vi "Set Instrument Addon Name.vi"(8 "Error In":errorcluster, 10 "Name":string="Instrument Addon", 11 "Instrument Addon Refnum In":T1 format="%.0x") -> (0 "Error Out":errorcluster, 3 "Instrument Addon Refnum Out":T1=18446744073709551615 format="%.0x")   [LabVIEW 2018, in "Instrument Addon Scripting API.lvlib"]
uses:
  Instrument Addon Scripting API.lvlib
  <vilib>/NI Veristand/Custom Device API/Custom Device Item Ref.ctl
  NationalInstruments.VeriStand.SystemDefinitionAPI
  NationalInstruments.VeriStand.SystemStorage
  Addon/Addon Shared/SubVIs/Constants.vi
  <vilib>/NI/NI VeriStand Advanced SysDef API/_SubVIs/SysDef.Search.GUIDs.vi
  <vilib>/NI Veristand/Custom Device Tools/Custom Device Utility Library/Custom Device Utility Library.lvlib
  <vilib>/NI/NI VeriStand Advanced SysDef API/SysDef API/Advanced System Definition.lvlib
  Addon/Addon Shared/Instrument Addon Shared.lvlib
  <vilib>/NI Veristand/Custom Device API/Custom Device API.lvlib
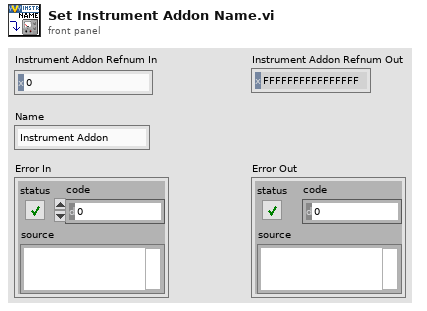
[diagram p1: front panel]
types:
  T1 = typedef "Custom Device API.lvlib/Custom Device Item Ref.ctl" = u64
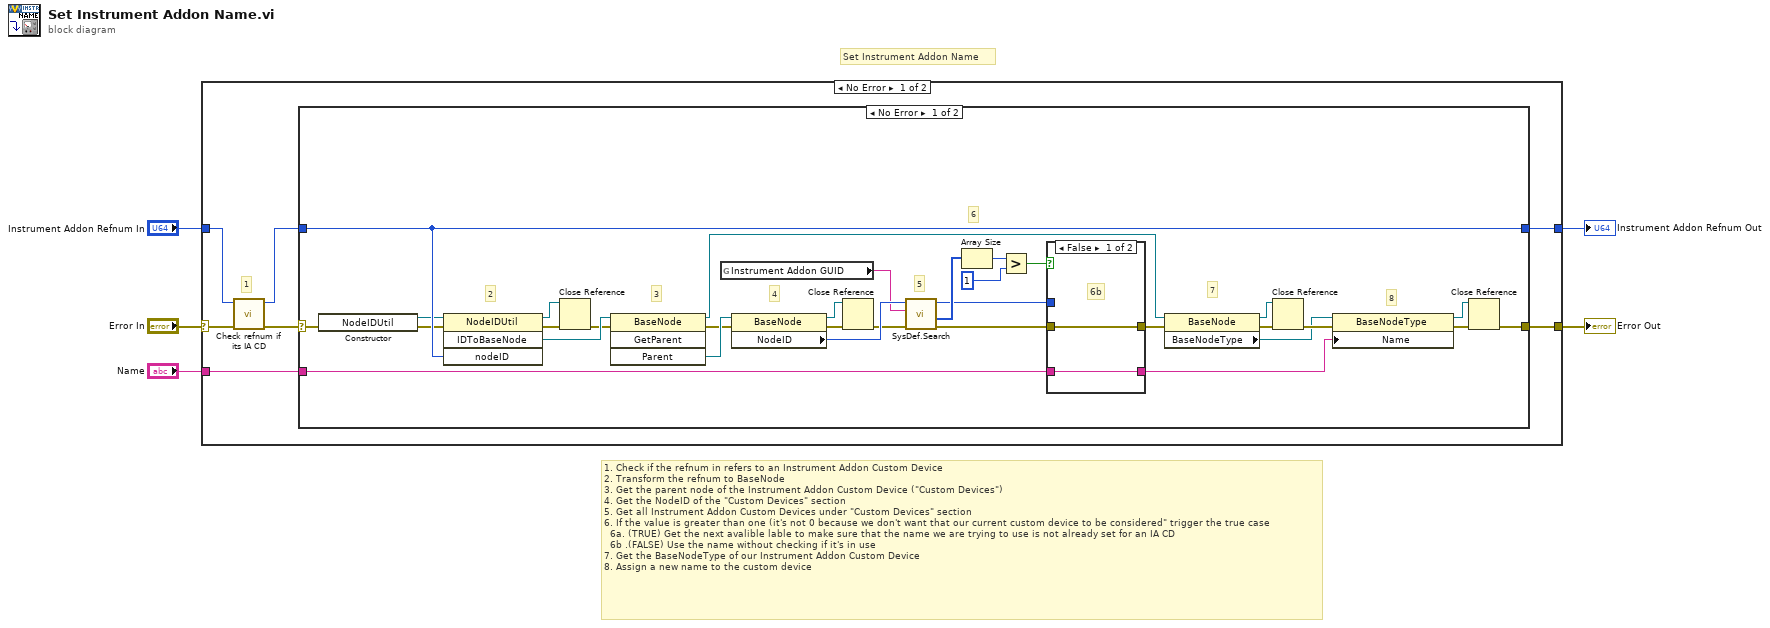
[diagram p0: block diagram]
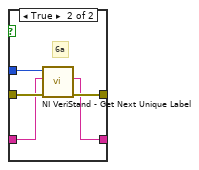
[diagram p2: hidden frame]
diagram:
  # "1. Check if the refnum in refers to an Instrument Addon Custom Device\n2. Transform the refnum to BaseNode\n3. Get the parent node of the Instrument Addon Custom Device (\"Custom Devices\")\n4. Get the NodeID of the \"Custom Devices\" section\n5. Get all Instrument Addon Custom Devices under \"Custom Devices\" section\n6. If the value is greater than one (it's not 0 because we don't want that our current custom device to be considered\" trigger the true case\n  6a. (TRUE) Get the next avalible lable to make sure that the name we are trying to use is not already set for an IA CD\n  6b .(FALSE) Use the name without checking if it's in use\n7. Get the BaseNodeType of our Instrument Addon Custom Device\n8. Assign a new name to the custom device"
  # "Set Instrument Addon Name"
  n1 = case shown="No Error" "Error In" {
    selector: "Error In" -> [w11 w55]
    tunnel: "Instrument Addon Refnum In" -> [w12 w54]
    tunnel: [w9 w55] -> w4
    tunnel: [w8 w54] -> w2
    tunnel: "Name" -> [w6 _]
    frame No Error {
      # "1"
      n2 = call "Check refnum if its IA CD.vi"("Error In"=w11, "Refnum In"=w12) -> ("Error Out"=w7:errorcluster, "Refnum Out"=w10:u64)  [unwired: 7 in, 1 out]
      n3 = case shown="No Error" w7 {
        selector: w7 -> [w42 w53]
        tunnel: w10 -> [w43 w52]
        tunnel: [w44 w53] -> w9
        tunnel: [w43 w52] -> w8
        tunnel: w6 -> [w41 _]
        frame No Error {
          # "8"
          # "7"
          # "6"
          # "5"
          # "4"
          # "3"
          # "2"
          n4 = constructor class="NodeIDUtil"(error in=w42) -> (reference out=w39:refnum<k24>, error out=w40:errorcluster)  [unwired: 2 in, 1 out]
          n5 = invoke class="NodeIDUtil" method="IDToBaseNode"(reference=w39, error in=w40, "nodeID"=w43) -> (reference out=w24:refnum<k24>, error out=w25:errorcluster, "IDToBaseNode"=w38:refnum<k24>)  [unwired: 1 in, 1 out]
          n6 = Close Reference(reference=w24, error in (no error)=w25) -> (error out=w23:errorcluster)
          n7 = invoke class="BaseNode" method="GetParent"(reference=w38, error in=w23) -> (reference out=w21:refnum<k24>, error out=w22:errorcluster, "Parent"=w37:refnum<k24>)  [unwired: 2 in, 1 out]
          n8 = global read "Constants.vi" "Instrument Addon GUID"() -> (w32:string)
          n9 = property class="BaseNode"(reference=w37, error in=w22) -> (reference out=w35:refnum<k24>, error out=w36:errorcluster, "NodeID"=w34:u64)
          n10 = Close Reference(reference=w35, error in (no error)=w36) -> (error out=w33:errorcluster)
          n11 = call-poly <vilib>:"SysDef.Search.vi"("error in (no error)"=w33, "GUID"=w32, "nodeID"=w34) -> ("error out"=w27:errorcluster, "Values Out"=w31:u64[], "nodeID out"=w26:u64)  [unwired: 5 in, 1 out]
          n12 = Array Size(array=w31) -> (size(s)=w30:i32)
          n13 = Greater?(x=w30, y=1) -> (0:w28:bool)
          n14 = case shown="False" w28 {
            tunnel: w27 -> [w46 w51]
            tunnel: w41 -> [w45 w50]
            tunnel: [w46 w49] -> w20
            tunnel: w26 -> [_ w48]
            tunnel: [w45 w47] -> w19
            frame False {
              # "6b"
            }
            frame True {
              # "6a"
              n15 = call <vilib>:"NI VeriStand - Get Next Unique Label.vi"("error in (no error)"=w51, "Label"=w50, "Parent Ref in"=w48) -> ("error out"=w49:errorcluster, "Label out"=w47:string)  [unwired: 5 in, 2 out]
            }
          }
          n16 = property class="BaseNode"(reference=w21, error in=w20) -> (reference out=w16:refnum<k24>, error out=w18:errorcluster, "BaseNodeType"=w15:refnum<k24>)
          n17 = Close Reference(reference=w16, error in (no error)=w18) -> (error out=w17:errorcluster)
          n18 = property class="BaseNodeType"(reference=w15, error in=w17, "Name"=w19) -> (reference out=w13:refnum<k24>, error out=w14:errorcluster)
          n19 = Close Reference(reference=w13, error in (no error)=w14) -> (error out=w44:errorcluster)
        }
        frame Error {
        }
      }
    }
    frame Error {
    }
  }
  "Error Out" <- w4
  "Instrument Addon Refnum Out" <- w2
